vi "Write Deposition status.vi"(8 "error in (no error)":errorcluster, 10 "Deposition status":string, 11 "SC-Main in":refnum<class "SC-Main.lvclass">) -> (0 "error out":errorcluster, 3 "SC-Main out":refnum<class "SC-Main.lvclass">)   [LabVIEW 2013, in "SLMControl.lvlib" / "SC-Main.lvclass"]
uses:
  SC-Main.lvclass
  SC-Main.lvclass/SC-Main.ctl
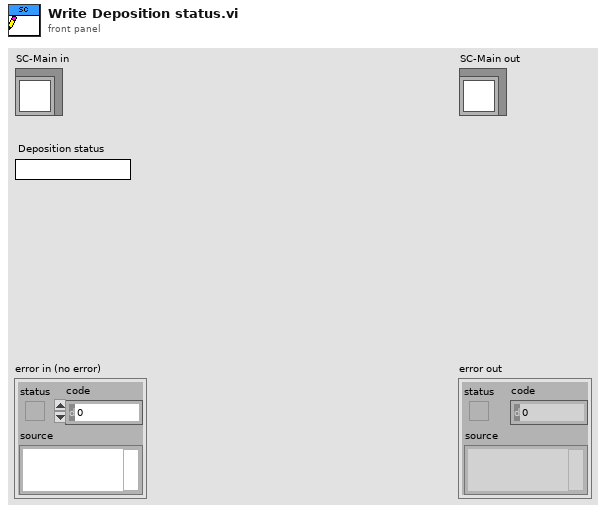
[diagram p1: front panel]
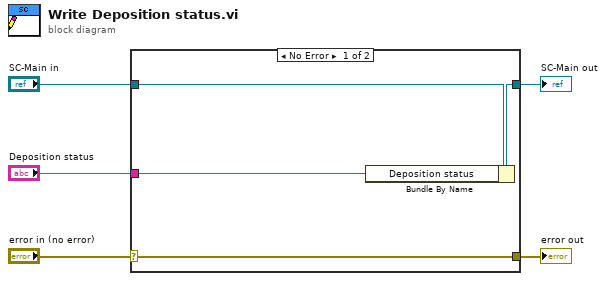
[diagram p0: block diagram]
diagram:
  n1 = case shown="No Error" "error in (no error)" {
    selector: "error in (no error)" -> [w9 w10]
    tunnel: [w9 w10] -> w4
    tunnel: [w7 w11] -> w2
    tunnel: "SC-Main in" -> [w8 w11]
    tunnel: "Deposition status" -> [w6 _]
    frame No Error {
      n2 = Bundle By Name(cluster=w8, "Deposition status"=w6) -> (w7:refnum<class "SC-Main.lvclass">)
    }
    frame Error {
    }
  }
  "error out" <- w4
  "SC-Main out" <- w2
